vi "write channel list to top file.vi"(8 "error in (no error)":errorcluster, 10 "ChannelList":T2, 11 "Refnum in":T1) -> (0 "error out":errorcluster, 3 "Refnum out":T1)   [LabVIEW 2015, in "SLSC Switch.lvlib" / "SLSC Switch.lvclass"]
uses:
  SLSC Switch.lvclass
  Controls/JSON.ChannelList.ctl
  <vilib>/Utility/config.llb/Config Data RefNum.ctl
  <vilib>/Utility/config.llb/NI_LVConfig.lvlib
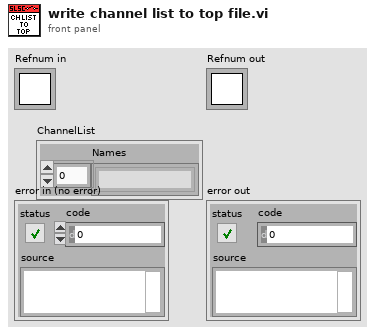
[diagram p1: front panel]
types:
  T1 = typedef "NI_LVConfig.lvlib/Config Data RefNum.ctl" = refnum<k1>
  T2 = typedef "SLSC Switch.lvlib/SLSC Switch.lvclass/JSON.ChannelList.ctl" = cluster{"Names":string[]}
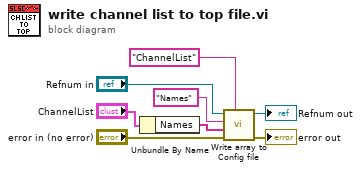
[diagram p0: block diagram]
diagram:
  n1 = Unbundle By Name("ChannelList") -> ("Names"=w1:string[])
  n2 = call "Write array to Config file.vi"("section"="ChannelList", "error in (no error)"="error in (no error)", "Array"=w1, "key"="Names", "Refnum in"="Refnum in") -> ("error out"=→"error out":errorcluster, "refnum out"=→"Refnum out":T1)  [unwired: 5 in]
